vi "数据处理.vi"() -> ()   [LabVIEW 2021]
uses:
  LabView Lib/QueueLib/QueueLib.lvlib
  a675053f-11e3-4344-be01-789a155e9c0b.vi
  9edb662d-976b-4785-95ef-1347320b0749.vi
  18077f71-1691-46fc-a8c5-88af8d42cd68.vi
  8b5f7df7-e831-4bb2-bc67-72ff672093b4.vi
panel:
  in  "显示所有曲线":bool=TRUE
  out "扫描代码":i16
  out "功能选择":enum32{"扫描", "脉冲", "维持时间"}(tab)
  out "扫描":T1 {"测试参数"."反向极限电流(mA)" min=0.0 max=3000.0; "测试参数"."反向电压(V)" min=-40.0 max=40.0; "测试参数"."正向极限电流(mA)" min=0.0 max=3000.0; "测试参数"."正向电压(V)" min=-40.0 max=40.0; "时序参数"."反改变量(V)" min=0.0 max=40.0 step=5e-06; "时序参数"."正改变量(V)" min=0.0 max=40.0 step=5e-06; "时序参数"."nplc" min=0.001}
  out "脉冲":T2 {"测试参数"."反向极限电流(mA)" min=0.0 max=3000.0; "测试参数"."反向电压(V)" min=-40.0 max=40.0; "测试参数"."读取电压(V)" min=-40.0 max=40.0; "测试参数"."正向极限电流(mA)" min=0.0 max=3000.0; "测试参数"."正向电压(V)" min=-40.0 max=40.0}
  out "维持时间":T3 {"时序参数"."nplc" min=0.001; "测试参数"."极限电流(mA)" min=0.0 max=3000.0; "测试参数"."读取电压(V)" min=-40.0 max=40.0}
  out "突变电压":dbl
  in  "删除":bool
  out "索引":i32 min=0 max=6
  in  "曲线设置":T4={"X轴数据选择"=enum."设置电压", "Y轴组"=[enum."读取电流"]}
  out "XY图":cluster{"测试数据":dbl[], "测试数据":dbl[]}[](graph)
  in  "测试类型":enum16{"扫描", "脉冲", "维持时间", "删除"}(ring)
  in  "打开数据":bool
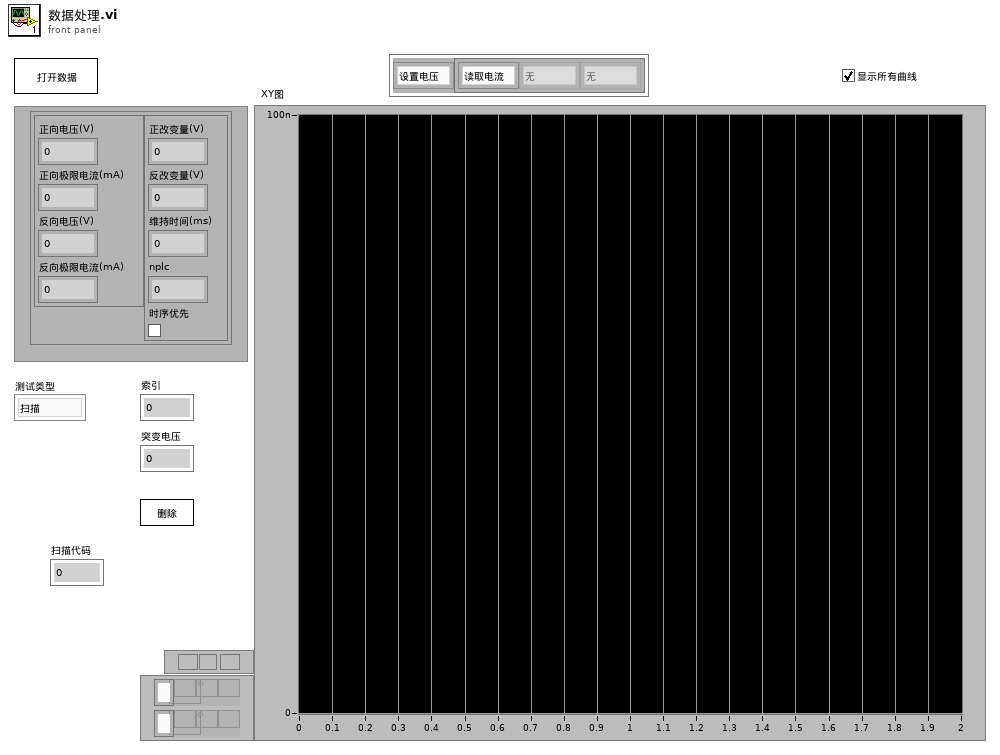
[diagram p1: front panel]
types:
  T1 = typedef "扫描参数.ctl" = cluster{"测试参数":cluster{"正向电压(V)":dbl, "正向极限电流(mA)":dbl, "反向电压(V)":dbl, "反向极限电流(mA)":dbl}, "时序参数":cluster{"正改变量(V)":dbl, "反改变量(V)":dbl, "维持时间(ms)":dbl, "nplc":dbl, "时序优先":bool}}
  T2 = typedef "脉冲参数.ctl" = cluster{"测试参数":cluster{"正向电压(V)":dbl, "正向极限电流(mA)":dbl, "反向电压(V)":dbl, "反向极限电流(mA)":dbl, "读取电压(V)":dbl}, "时序参数":cluster{"脉冲宽度(ms)":dbl, "读取次数":u32}}
  T3 = typedef "维持时间.ctl" = cluster{"测试参数":cluster{"读取电压(V)":dbl, "极限电流(mA)":dbl}, "时序参数":cluster{"测试时间(s)":dbl, "读取间隔(ms)":dbl, "nplc":dbl, "时序优先":bool}}
  T4 = typedef "曲线设置.ctl" = cluster{"X轴数据选择":enum16{"时间", "设置电压", "读取电流", "读取电压"}, "Y轴组":enum16{"时间", "设置电压", "读取电流", "读取电压", "无"}[]}
  T5 = typedef "测试数据类型.ctl" = cluster{"测试时间":timestamp, "数据":dbl[][], "功能":string, "方向":string, "循环":bool, "样品标记":string, "突变电压":i32, "所属tdms":refnum<k34>, "组名称":string, "删除":bool, "测试参数":string}
  T6 = typedef "缓冲数据.ctl" = cluster{"扫描":T5[], "脉冲":T5[], "维持时间":T5[], "删除":T5[]}
  T7 = typedef "QueueLib.lvlib/数据类型.ctl" = cluster{"消息":string, "数据":variant}
  T8 = typedef "曲线属性.ctl" = cluster{"曲线名":string, "曲线颜色":u32}
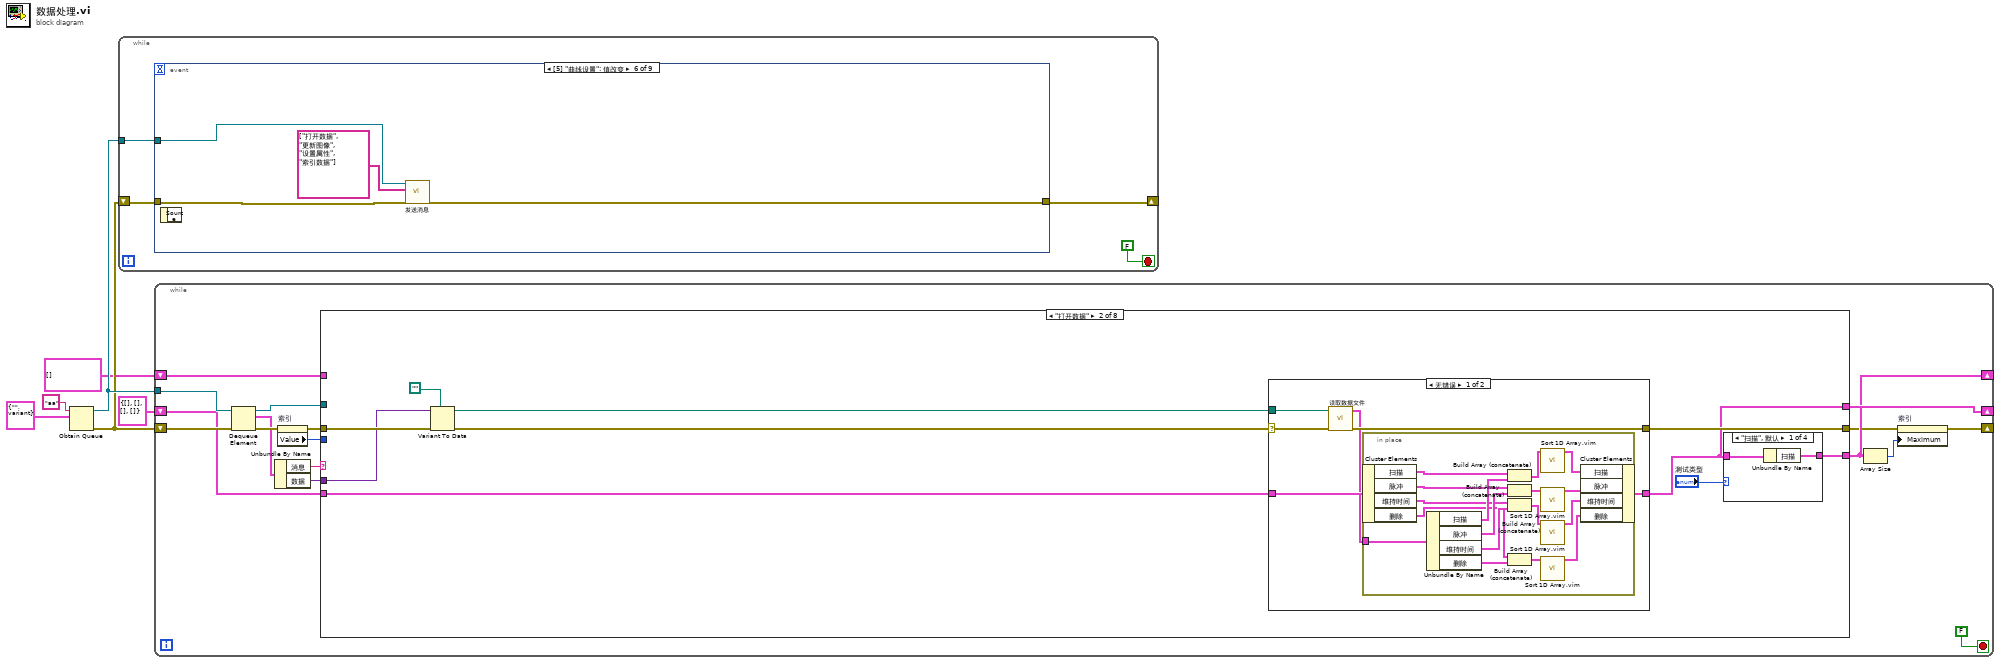
[diagram p0: block diagram]
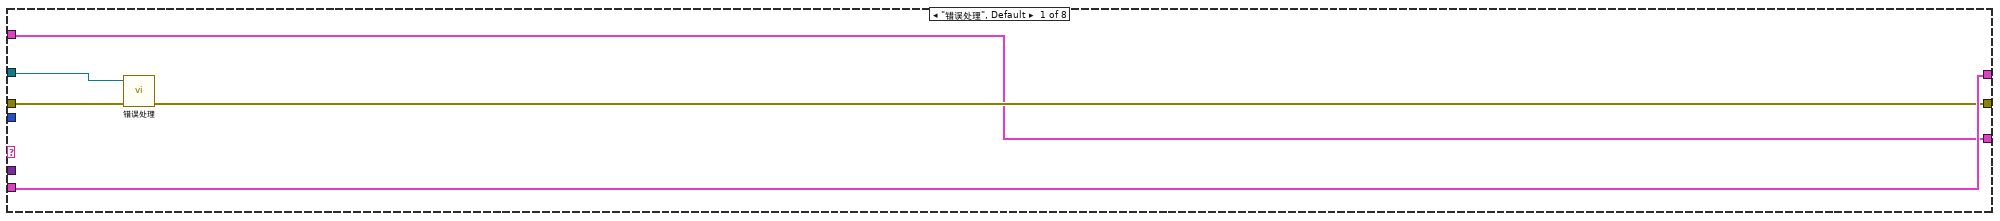
[diagram p2: hidden frame]
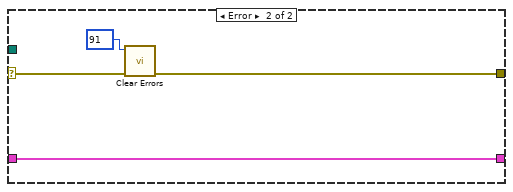
[diagram p3: hidden frame]
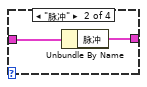
[diagram p4: hidden frame]
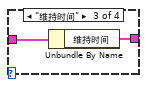
[diagram p5: hidden frame]
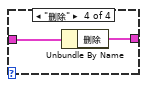
[diagram p6: hidden frame]
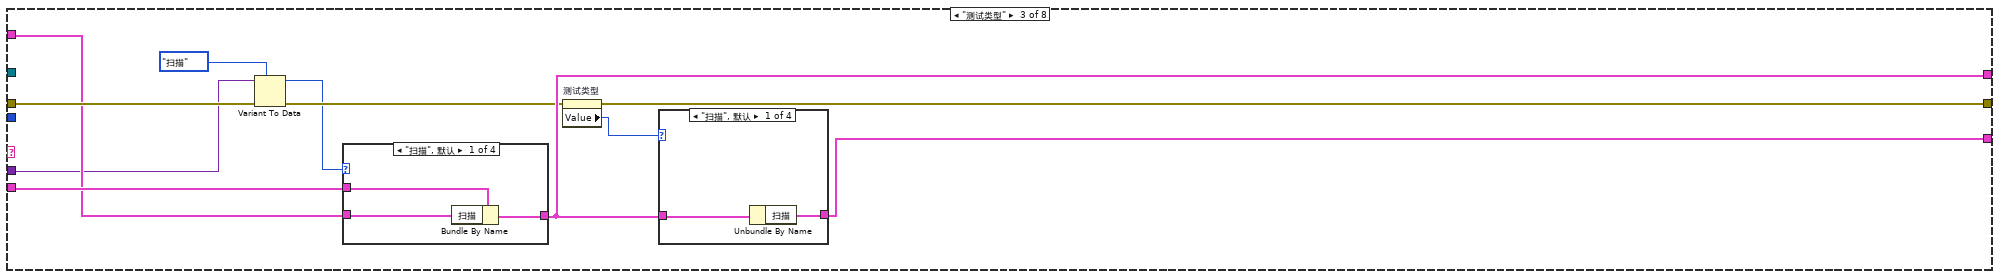
[diagram p7: hidden frame]
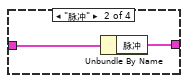
[diagram p8: hidden frame]
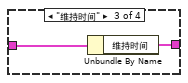
[diagram p9: hidden frame]
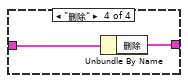
[diagram p10: hidden frame]
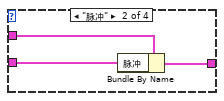
[diagram p11: hidden frame]
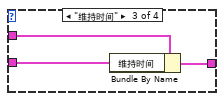
[diagram p12: hidden frame]
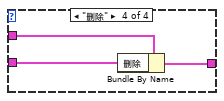
[diagram p13: hidden frame]
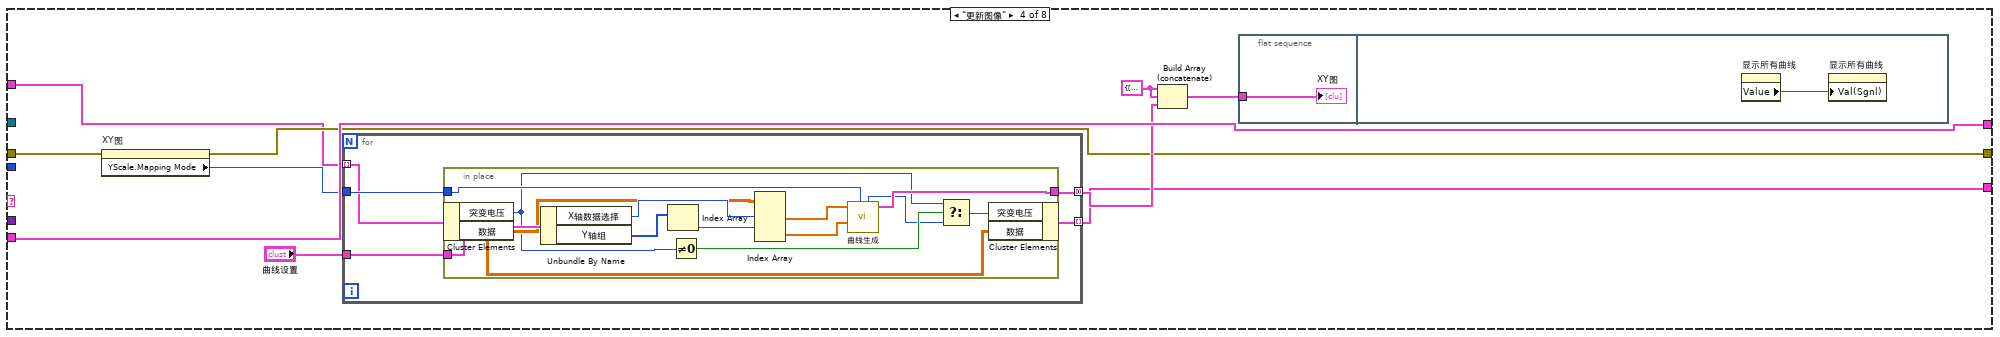
[diagram p14: hidden frame]
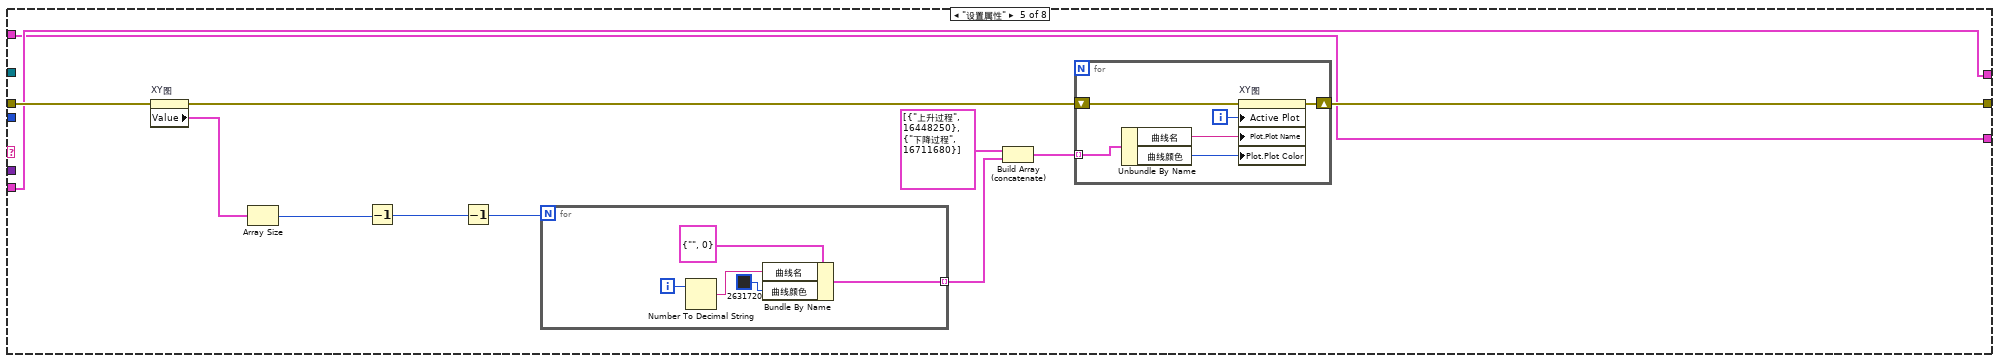
[diagram p15: hidden frame]
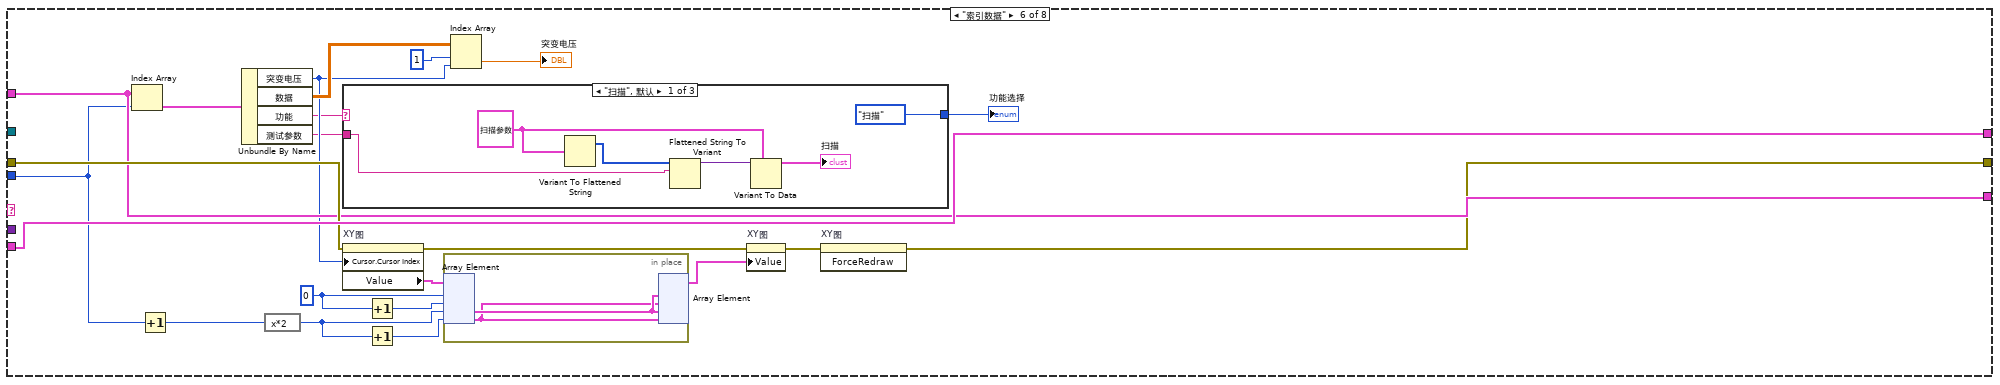
[diagram p16: hidden frame]
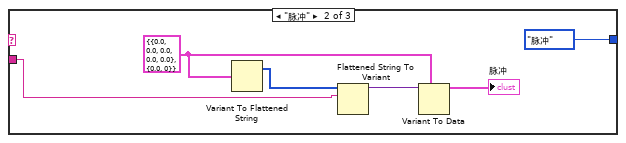
[diagram p17: hidden frame]
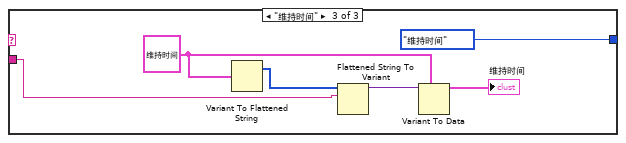
[diagram p18: hidden frame]
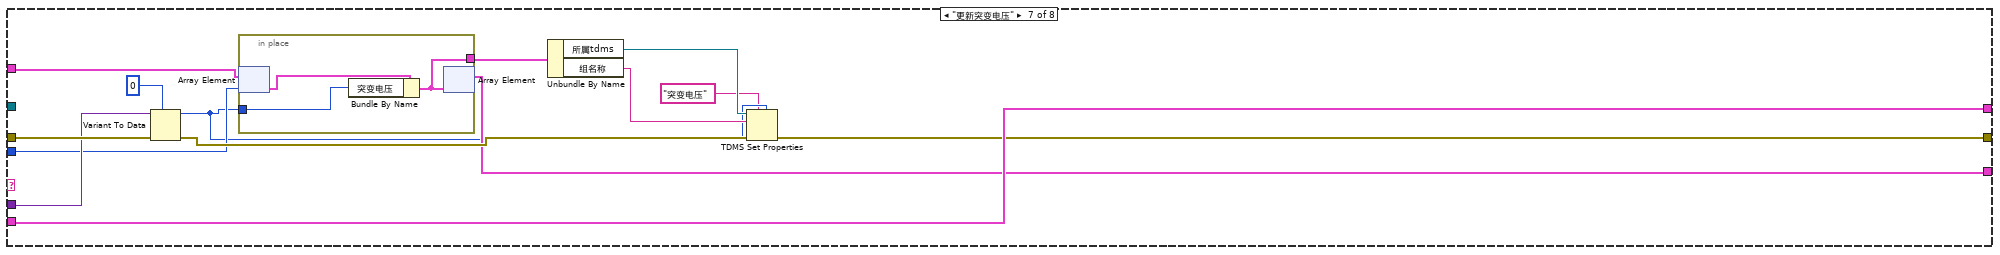
[diagram p19: hidden frame]
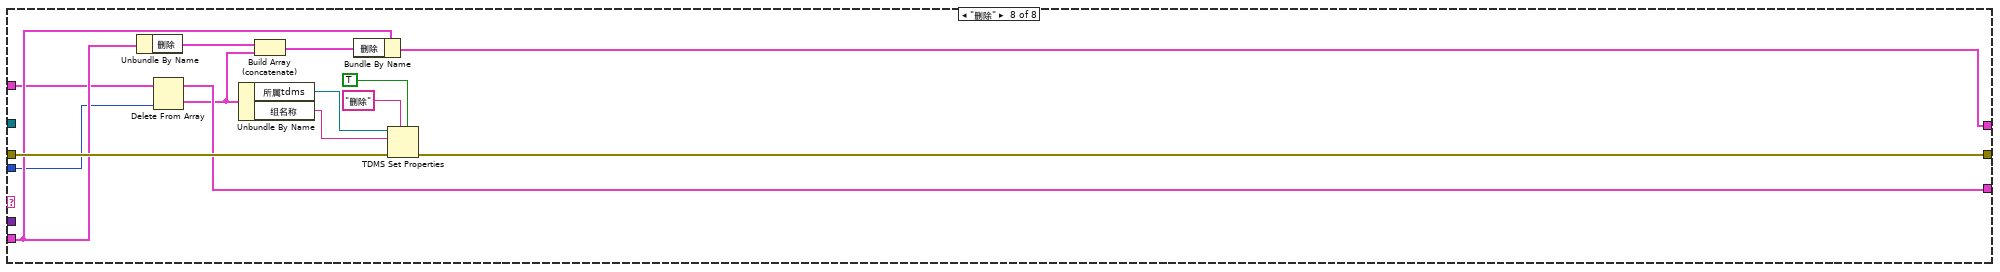
[diagram p20: hidden frame]
diagram:
  n1 = Obtain Queue(name (unnamed)="aa" ("名称（未命名）"), element data type=T7 {"消息"="", "数据"=variant} ("数据类型")) -> (queue out=w4:refnum<queue>, error out=w3:errorcluster)  [unwired: 3 in, 1 out]
  n2 = while {
    tunnel: w4 -> [w9]
    shift-right: [w7] -> _
    shift-left: w3 -> [w8]
    stop <- FALSE stop-if-true
    n3 = event shown="[5] \"曲线设置\": 值改变" {
      selector: _ -> [_ _ _ _ _ _ _ _ _]
      dyn-events: _ -> [_ _ _ _ _ _ _ _ _]
      timeout: _ -> [_ _ _ _ _ _ _ _ _]
      tunnel: w9 -> [w18 w20 _ w53 w55 w61 _ w73 w77]
      tunnel: w8 -> [w16 w22 w47 w52 w57 w59 w66 w75 w79]
      tunnel: [w19 w21 w47 w51 w56 w60 w66 w74 w78] -> w7
      event "打开数据": Value Change {
        n4 = event-data() -> ()  [unwired: 1 in, 1 out]
        n5 = call "文件对话框"("start path"=path "D:/Data", "error in"=w16) -> ("selected path"=w13:path, "error out"=w15:errorcluster)  [unwired: 10 in, 2 out]
        n6 = To Variant(anything=w13) -> (Variant=w12:variant)
        n7 = Build Array(w12) -> (w11:variant[])
        n8 = call-poly "发送消息.vi"("错误输入（无错误）"=w15, "数据列表"=w11, "消息列表"=string[] ["打开数据", "更新图像", "设置属性", "索引数据"], "输入队列"=w18) -> ("错误输出"=w19:errorcluster)  [unwired: 6 in, 1 out]
      }
      event Key Down {
        n9 = event-data() -> ("ScanCode"=w23:i16)  [unwired: 1 in]
        n10 = case shown="72, 80" w23 {
          selector: w23 -> [_ w29 _]
          tunnel: w22 -> [w24 w33 w44]
          tunnel: [w24 w31 w43] -> w21
          tunnel: w20 -> [_ _ w42]
          frame 0, Default {
          }
          frame 72, 80 {
            n11 = property on="索引" class="DigNum (严格)"(error in=w33) -> (error out=w32:errorcluster, "Value"=w30:i32, "Maximum"=w28:dbl, "Minimum"=w27:dbl)  [unwired: 1 in, 1 out]
            n12 = case shown="72" w29 {
              tunnel: w30 -> [w39 w41]
              tunnel: [w38 w40] -> w26
              frame Default {
                n13 = Decrement(x=w39) -> (x-1=w38:i32)
              }
              frame 72 {
                n14 = Increment(x=w41) -> (x+1=w40:i32)
              }
            }
            n15 = In Range and Coerce(upper limit=w28, x=w26, lower limit=w27) -> (In Range?=w25:bool)  [unwired: 1 out]
            n16 = case shown="假" w25 {
              tunnel: w32 -> [w34 w37]
              tunnel: [w34 w36] -> w31
              tunnel: w26 -> [_ w35]
              frame False {
              }
              frame True {
                n17 = property on="索引" class="DigNum (严格)"(error in=w37, "Val(Sgnl)"=w35) -> (error out=w36:errorcluster)  [unwired: 1 in, 1 out]
              }
            }
          }
          frame 83 {
            n18 = call-poly "发送消息.vi"("错误输入（无错误）"=w44, "消息列表"=string[] ["删除", "更新图像", "索引数据"], "输入队列"=w42) -> ("错误输出"=w43:errorcluster)  [unwired: 7 in, 1 out]
          }
        }
      }
      event Key Repeat {
        n19 = event-data() -> ("ScanCode"=→"扫描代码":i16)  [unwired: 1 in]
      }
      event "测试类型": Value Change {
        n20 = event-data() -> ("OldVal"=w49:enum16{"扫描", "脉冲", "维持时间", "删除"})  [unwired: 1 in]
        n21 = Build Array(w49) -> (w48:enum16{"扫描", "脉冲", "维持时间", "删除"}[])
        n22 = call-poly "发送消息.vi"("错误输入（无错误）"=w52, "数据列表"=w48, "消息列表"=string[] ["测试类型", "更新图像", "设置属性", "索引数据"], "输入队列"=w53) -> ("错误输出"=w51:errorcluster)  [unwired: 6 in, 1 out]
      }
      event "索引": Value Change {
        n23 = event-data() -> ()  [unwired: 1 in, 1 out]
        n24 = call-poly "发送消息.vi"("错误输入（无错误）"=w57, "消息"="索引数据", "输入队列"=w55) -> ("错误输出"=w56:errorcluster)  [unwired: 7 in, 1 out]
      }
      event Value Change {
        n25 = event-data() -> ()  [unwired: 1 in, 1 out]
        n26 = call-poly "发送消息.vi"("错误输入（无错误）"=w59, "消息列表"=string[] ["打开数据", "更新图像", "设置属性", "索引数据"], "输入队列"=w61) -> ("错误输出"=w60:errorcluster)  [unwired: 7 in, 1 out]
      }
      event "显示所有曲线": Value Change {
        n27 = event-data() -> ()  [unwired: 1 in, 2 out]
        n28 = property on="XY图" class="XYGraph (严格)"() -> ("Value"=w65:cluster{"测试数据":dbl[], "测试数据":dbl[]}[])  [unwired: 2 in, 2 out]
        n29 = Array Size(array=w65) -> (size(s)=w64:i32)
        n30 = expression code="x-2"(w64) -> (w63:i32)
        n31 = for {
          N: w63 -> [_]
          tunnel: "显示所有曲线" -> [w67]
          i -> [w69]
          n32 = expression code="x+2"(w69) -> (w68:i32)
          n33 = property on="XY图" class="XYGraph (严格)"("Active Plot"=w68, "Plot.Visible?"=w67) -> ()  [unwired: 2 in, 2 out]
        }
      }
      event "XY图": Cursor Release {
        n34 = event-data() -> ("PointIdx"=w72:i32)  [unwired: 1 in]
        n35 = Build Array(w72) -> (w70:i32[])
        n36 = call-poly "发送消息.vi"("错误输入（无错误）"=w75, "数据列表"=w70, "消息列表"=string[] ["更新突变电压", "索引数据"], "输入队列"=w73) -> ("错误输出"=w74:errorcluster)  [unwired: 6 in, 1 out]
      }
      event "删除": Value Change {
        n37 = event-data() -> ()  [unwired: 1 in, 1 out]
        n38 = call-poly "发送消息.vi"("错误输入（无错误）"=w79, "消息列表"=string[] ["删除", "更新图像", "索引数据"], "输入队列"=w77) -> ("错误输出"=w78:errorcluster)  [unwired: 7 in, 1 out]
      }
    }
  }
  n39 = while {
    tunnel: w4 -> [w96]
    shift-right: [w80] -> _
    shift-left: w3 -> [w95]
    shift-right: [w91] -> _
    shift-left: T6 {"扫描"=[], "脉冲"=[], "维持时间"=[], "删除"=[]} ("数据") -> [w90]
    shift-right: [w83] -> _
    shift-left: T5[] [] ("维持时间") -> [w86]
    stop <- FALSE stop-if-true
    n40 = Dequeue Element(queue=w96, error in (no error)=w95) -> (queue out=w87:refnum<queue>, element=w93:T7, error out=w94:errorcluster)  [unwired: 1 in, 1 out]
    n41 = Unbundle By Name(w93) -> ("消息"=w92:string, "数据"=w88:variant)
    n42 = property on="索引" class="DigNum (严格)"(error in=w94) -> (error out=w85:errorcluster, "Value"=w84:i32)  [unwired: 1 in, 1 out]
    n43 = case shown="\"打开数据\"" w92 {
      tunnel: w85 -> [w100 w110 w157 w181 w219 w246 w286 w303]
      tunnel: [w99 w111 w147 w180 w209 w238 w278 w297] -> w81
      tunnel: [w101 w107 w154 w187 w218 w252 w285 w298] -> w91
      tunnel: w90 -> [w101 w102 w156 w187 w218 w252 w285 w302]
      tunnel: w88 -> [_ w109 w151 _ _ _ w283 _]
      tunnel: w87 -> [w98 _ _ _ _ _ _ _]
      tunnel: [w97 w105 w148 w178 w208 w244 w279 w300] -> w83
      tunnel: w86 -> [w97 _ w155 w179 w208 w244 w281 w301]
      tunnel: w84 -> [_ _ _ _ _ w242 w280 w299]
      frame "错误处理", Default {
        n44 = call "错误处理.vi"("错误输入（无错误）"=w100, "队列输入"=w98) -> ("错误输出"=w99:errorcluster)  [unwired: 9 in]
      }
      frame "打开数据" {
        n45 = Variant To Data(error in=w110, type=path "", Variant=w109) -> (data=w106:path, error out=w104:errorcluster)
        n46 = case shown="无错误" w104 {
          selector: w104 -> [w115 w138]
          tunnel: [w117 w137] -> w111
          tunnel: w102 -> [w114 w135]
          tunnel: [w112 w135] -> w107
          tunnel: w106 -> [w116 _]
          frame No Error {
            n47 = call "读取数据文件.vi"("错误输入（无错误）"=w115, "tdms文件路径"=w116) -> ("错误输出"=w117:errorcluster, "数据"=w113:T6)  [unwired: 8 in]
            n48 = in-place {
              in-place-border: w113 -> [w126]
              n49 = in-place-cluster #1(w114) -> ("扫描"=w125:T5[], "脉冲"=w124:T5[], "维持时间"=w123:T5[], "删除"=w122:T5[])
              n50 = Unbundle By Name(w126) -> ("扫描"=w132:T5[], "脉冲"=w131:T5[], "维持时间"=w130:T5[], "删除"=w134:T5[])
              n51 = Build Array (concatenate)(w125, w132) -> (w129:T5[])
              n52 = Build Array (concatenate)(w124, w131) -> (w128:T5[])
              n53 = Build Array (concatenate)(w123, w130) -> (w127:T5[])
              n54 = Build Array (concatenate)(w122, w134) -> (w133:T5[])
              n55 = call "Sort 1D Array.vim"("unsorted array"=w129) -> ("sorted array"=w121:T5[])  [unwired: 10 in]
              n56 = call "Sort 1D Array.vim"("unsorted array"=w128) -> ("sorted array"=w120:T5[])  [unwired: 10 in]
              n57 = call "Sort 1D Array.vim"("unsorted array"=w127) -> ("sorted array"=w119:T5[])  [unwired: 10 in]
              n58 = call "Sort 1D Array.vim"("unsorted array"=w133) -> ("sorted array"=w118:T5[])  [unwired: 10 in]
              n59 = in-place-cluster #1("扫描"=w121, "脉冲"=w120, "维持时间"=w119, "删除"=w118) -> (w112:T6)
            }
          }
          frame Error {
            n60 = call <vilib>:"Clear Errors.vi"("error in (no error)"=w138, "specific error code to clear (0: all)"=91) -> ("error out"=w137:errorcluster)  [unwired: 4 in, 1 out]
          }
        }
        n61 = case shown="\"扫描\", 默认" "测试类型" {
          tunnel: w107 -> [w140 w142 w144 w146]
          tunnel: [w139 w141 w143 w145] -> w105
          frame "扫描", Default {
            n62 = Unbundle By Name(w140) -> ("扫描"=w139:T5[])
          }
          frame "脉冲" {
            n63 = Unbundle By Name(w142) -> ("脉冲"=w141:T5[])
          }
          frame "维持时间" {
            n64 = Unbundle By Name(w144) -> ("维持时间"=w143:T5[])
          }
          frame "删除" {
            n65 = Unbundle By Name(w146) -> ("删除"=w145:T5[])
          }
        }
      }
      frame "测试类型" {
        n66 = Variant To Data(error in=w157, type=enum16{"扫描", "脉冲", "维持时间", "删除"}."扫描" ("测试类型"), Variant=w151) -> (data=w149:enum16{"扫描", "脉冲", "维持时间", "删除"}, error out=w152:errorcluster)
        n67 = case shown="\"扫描\", 默认" w149 {
          tunnel: w156 -> [w167 w171 w174 w177]
          tunnel: [w166 w170 w173 w176] -> w154
          tunnel: w155 -> [w168 w169 w172 w175]
          frame "扫描", Default {
            n68 = Bundle By Name(cluster=w167, "扫描"=w168) -> (w166:T6)
          }
          frame "脉冲" {
            n69 = Bundle By Name(cluster=w171, "脉冲"=w169) -> (w170:T6)
          }
          frame "维持时间" {
            n70 = Bundle By Name(cluster=w174, "维持时间"=w172) -> (w173:T6)
          }
          frame "删除" {
            n71 = Bundle By Name(cluster=w177, "删除"=w175) -> (w176:T6)
          }
        }
        n72 = property on="测试类型" class="Enum (严格)"(error in=w152) -> (error out=w147:errorcluster, "Value"=w153:enum16{"扫描", "脉冲", "维持时间", "删除"})  [unwired: 1 in, 1 out]
        n73 = case shown="\"扫描\", 默认" w153 {
          tunnel: w154 -> [w159 w161 w163 w165]
          tunnel: [w158 w160 w162 w164] -> w148
          frame "扫描", Default {
            n74 = Unbundle By Name(w159) -> ("扫描"=w158:T5[])
          }
          frame "脉冲" {
            n75 = Unbundle By Name(w161) -> ("脉冲"=w160:T5[])
          }
          frame "维持时间" {
            n76 = Unbundle By Name(w163) -> ("维持时间"=w162:T5[])
          }
          frame "删除" {
            n77 = Unbundle By Name(w165) -> ("删除"=w164:T5[])
          }
        }
      }
      frame "更新图像" {
        w182 = cluster{dbl[], dbl[]} {[0.0], [0.0]}
        n78 = property on="XY图" class="XYGraph (严格)"(error in=w181) -> (error out=w180:errorcluster, "YScale.Mapping Mode"=w186:u8)  [unwired: 1 in, 1 out]
        n79 = for {
          tunnel: w186 -> [w194]
          tunnel: w179 -> [w191] mode=indexing
          tunnel: "曲线设置" -> [w193]
          tunnel: [w192] -> w184 mode=concatenating
          tunnel: [w190] -> w178 mode=indexing
          n80 = in-place {
            in-place-border: w194 -> [w207]
            in-place-border: w193 -> [w203]
            in-place-border: [w200] -> w192
            n81 = in-place-cluster #2(w191) -> ("突变电压"=w196:i32, "数据"=w199:dbl[][])
            n82 = Unbundle By Name(w203) -> ("X轴数据选择"=w205:enum16{"时间", "设置电压", "读取电流", "读取电压"}, "Y轴组"=w204:enum16{"时间", "设置电压", "读取电流", "读取电压", "无"}[])
            n83 = Index Array(array=w204) -> (element=w206:enum16{"时间", "设置电压", "读取电流", "读取电压", "无"})  [unwired: 1 in]
            n84 = Not Equal To 0?(x=w196) -> (x != 0?=w198:bool)
            n85 = Index Array(array=w199, index (row) #1=w205, index (row) #2=w206) -> (element #1=w202:dbl[], element #2=w201:dbl[])  [unwired: 2 in]
            n86 = call "曲线生成.vi"("YScale.Mapping Mode"=w207, "Y"=w201, "X"=w202) -> ("曲线"=w200:cluster{dbl[], dbl[]}[], "突变电压"=w197:i32)  [unwired: 7 in]
            n87 = Select(t=w196, s=w198, f=w197) -> (s? t:f=w195:i32)
            n88 = in-place-cluster #2("突变电压"=w195, "数据"=w199) -> (w190:T5)
          }
        }
        n89 = Build Array (concatenate)(w182, w182, w184) -> (w183:cluster{dbl[], dbl[]}[])
        n90 = flat-sequence {
          tunnel: w183 -> [w188]
          frame #0 {
            "XY图" <- w188
          }
          frame #1 {
            n91 = property on="显示所有曲线" class="Bool (严格)"() -> ("Value"=w189:bool)  [unwired: 2 in, 2 out]
            n92 = property on="显示所有曲线" class="Bool (严格)"("Val(Sgnl)"=w189) -> ()  [unwired: 2 in, 2 out]
          }
        }
      }
      frame "设置属性" {
        n93 = property on="XY图" class="XYGraph (严格)"(error in=w219) -> (error out=w210:errorcluster, "Value"=w214:cluster{"测试数据":dbl[], "测试数据":dbl[]}[])  [unwired: 1 in, 1 out]
        n94 = Array Size(array=w214) -> (size(s)=w213:i32)
        n95 = Decrement(x=w213) -> (x-1=w211:i32)
        n96 = Decrement(x=w211) -> (x-1=w212:i32)
        n97 = for {
          N: w212 -> [_]
          tunnel: [w226] -> w217 mode=indexing
          i -> [w227]
          n98 = Number To Decimal String(number=w227) -> (decimal integer string=w228:string)  [unwired: 1 in]
          n99 = Bundle By Name(cluster=T8 {"曲线名"="", "曲线颜色"=0} ("曲线属性"), "曲线名"=w228, "曲线颜色"=u32 2631720) -> (w226:T8)
        }
        n100 = Build Array (concatenate)(T8[] [{"曲线名"="上升过程", "曲线颜色"=16448250}, {"曲线名"="下降过程", "曲线颜色"=16711680}], w217) -> (w215:T8[])
        n101 = for {
          tunnel: w215 -> [w223] mode=indexing
          shift-right: [w220] -> w209
          shift-left: w210 -> [w221]
          i -> [w225]
          n102 = Unbundle By Name(w223) -> ("曲线名"=w224:string, "曲线颜色"=w222:u32)
          n103 = property on="XY图" class="XYGraph (严格)"(error in=w221, "Active Plot"=w225, "Plot.Plot Name"=w224, "Plot.Plot Color"=w222) -> (error out=w220:errorcluster)  [unwired: 1 in, 1 out]
        }
      }
      frame "索引数据" {
        w248 = 0
        n104 = Index Array(array=w244, index=w242) -> (element=w243:T5)
        n105 = Increment(x=w242) -> (x+1=w241:i32)
        n106 = Unbundle By Name(w243) -> ("突变电压"=w236:i32, "数据"=w237:dbl[][], "功能"=w233:string, "测试参数"=w231:string)
        n107 = expression code="x*2"(w241) -> (w250:i32)
        n108 = case shown="\"扫描\", 默认" w233 {
          tunnel: [enum32{"扫描", "脉冲", "维持时间"}."扫描" ("功能选择") enum32{"扫描", "脉冲", "维持时间"}."脉冲" ("功能选择") enum32{"扫描", "脉冲", "维持时间"}."维持时间" ("功能选择")] -> w232
          tunnel: w231 -> [w253 w261 w267]
          frame "扫描", Default {
            w254 = T1 {"测试参数"={"正向电压(V)"=0.0, "正向极限电流(mA)"=0.0, "反向电压(V)"=0.0, "反向极限电流(mA)"=0.0}, "时序参数"={"正改变量(V)"=0.0, "反改变量(V)"=0.0, "维持时间(ms)"=0.0, "nplc"=0.0, "时序优先"=FALSE}} ("扫描")
            n109 = Variant To Flattened String(Variant=w254) -> (1:w257:i16[])  [unwired: 1 out]
            n110 = Flattened String To Variant(6:w253, 7:w257) -> (3:w256:variant)  [unwired: 1 in, 1 out]
            n111 = Variant To Data(type=w254, Variant=w256) -> (data=→"扫描":T1)  [unwired: 1 in, 1 out]
          }
          frame "脉冲" {
            w260 = T2 {"测试参数"={"正向电压(V)"=0.0, "正向极限电流(mA)"=0.0, "反向电压(V)"=0.0, "反向极限电流(mA)"=0.0, "读取电压(V)"=0.0}, "时序参数"={"脉冲宽度(ms)"=0.0, "读取次数"=0}} ("脉冲")
            n112 = Variant To Flattened String(Variant=w260) -> (1:w263:i16[])  [unwired: 1 out]
            n113 = Flattened String To Variant(6:w261, 7:w263) -> (3:w262:variant)  [unwired: 1 in, 1 out]
            n114 = Variant To Data(type=w260, Variant=w262) -> (data=→"脉冲":T2)  [unwired: 1 in, 1 out]
          }
          frame "维持时间" {
            w265 = T3 {"测试参数"={"读取电压(V)"=0.0, "极限电流(mA)"=0.0}, "时序参数"={"测试时间(s)"=0.0, "读取间隔(ms)"=0.0, "nplc"=0.001, "时序优先"=FALSE}} ("数据")
            n115 = Variant To Flattened String(Variant=w265) -> (1:w269:i16[])  [unwired: 1 out]
            n116 = Flattened String To Variant(6:w267, 7:w269) -> (3:w268:variant)  [unwired: 1 in, 1 out]
            n117 = Variant To Data(type=w265, Variant=w268) -> (data=→"维持时间":T3)  [unwired: 1 in, 1 out]
          }
        }
        "功能选择" <- w232
        n118 = property on="XY图" class="XYGraph (严格)"(error in=w246, "Cursor.Cursor Index"=w236) -> (error out=w245:errorcluster, "Value"=w240:cluster{"测试数据":dbl[], "测试数据":dbl[]}[])  [unwired: 1 in, 1 out]
        n119 = Increment(x=w248) -> (x+1=w247:i32)
        n120 = Increment(x=w250) -> (x+1=w249:i32)
        n121 = in-place {
          n122 = in-place-array #3(w240, w248, w247, w250, w249) -> (w272:cluster{"测试数据":dbl[], "测试数据":dbl[]}, w271:cluster{"测试数据":dbl[], "测试数据":dbl[]})  [unwired: 2 out]
          n123 = in-place-array #3(w272, w271, w272, w271) -> (w251:cluster{"测试数据":dbl[], "测试数据":dbl[]}[])  [unwired: 4 out]
        }
        n124 = Index Array(array=w237, index (row)=1 ("禁用的索引 (行)"), index (col)=w236) -> (element=→"突变电压":dbl)
        n125 = property on="XY图" class="XYGraph (严格)"(error in=w245, "Value"=w251) -> (error out=w239:errorcluster)  [unwired: 1 in, 1 out]
        n126 = invoke on="XY图" class="XYGraph (严格)" method="ForceRedraw"(error in=w239) -> (error out=w238:errorcluster)  [unwired: 2 in, 2 out]
      }
      frame "更新突变电压" {
        n127 = Variant To Data(error in=w286, type=0, Variant=w283) -> (data=w274:i32, error out=w284:errorcluster)
        n128 = in-place {
          in-place-border: w274 -> [w288]
          in-place-border: [w287] -> w277
          n129 = in-place-array #4(w281, w280) -> (w289:T5)
          n130 = Bundle By Name(cluster=w289, "突变电压"=w288) -> (w287:T5)
          n131 = in-place-array #4(w287) -> (w279:T5[])  [unwired: 1 out]
        }
        n132 = Unbundle By Name(w277) -> ("所属tdms"=w276:refnum<k34>, "组名称"=w275:string)
        n133 = TDMS Set Properties(5:w274, 7:"突变电压" ("属性名称"), 8:w284, 10:w275, 11:w276) -> (0:w278:errorcluster)  [unwired: 1 in, 3 out]
      }
      frame "删除" {
        n134 = Unbundle By Name(w302) -> ("删除"=w291:T5[])
        n135 = Delete From Array(array=w301, index=w299) -> (deleted portion=w296:T5, array with subset deleted=w300:T5[])  [unwired: 1 in]
        n136 = Unbundle By Name(w296) -> ("所属tdms"=w295:refnum<k34>, "组名称"=w294:string)
        n137 = Build Array (concatenate)(w291, w296) -> (w290:T5[])
        n138 = Bundle By Name(cluster=w302, "删除"=w290) -> (w298:T6)
        n139 = TDMS Set Properties(5:TRUE, 7:"删除", 8:w303, 10:w294, 11:w295) -> (0:w297:errorcluster)  [unwired: 1 in, 3 out]
      }
    }
    n140 = Array Size(array=w83) -> (size(s)=w82:i32)
    n141 = property on="索引" class="DigNum (严格)"(error in=w81, "Maximum"=w82) -> (error out=w80:errorcluster)  [unwired: 1 in, 1 out]
  }
